vi "2898 Updated Secondary.vi"() -> (8 "Shooting Manual Override?":bool)   [LabVIEW 2011]
uses:
  Team Code/Robot Global Data.vi
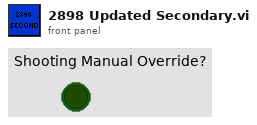
[diagram p1: front panel]
types:
  T1 = cluster{"Buttons":cluster{"A":bool, "B":bool, "X":bool, "Y":bool, "Left Bumper":bool, "Right Bumper":bool, "Back":bool, "Start":bool, "Left Thumbstick":bool, "Right Thumbstick":bool}, "Axes":cluster{"Left X ":dbl, "Left Y":dbl, "Triggers":dbl, "Right Stick X":dbl, "Right Stick Y":dbl, "D-Pad X":dbl}}
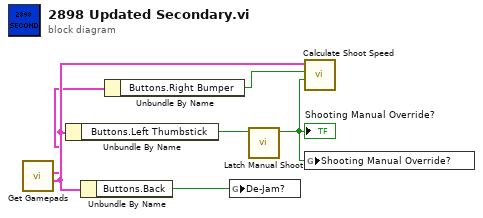
[diagram p0: block diagram]
diagram:
  n1 = call "Get Gamepads.vi"() -> ("Secondary"=w6:T1, "Driver"=w2:T1)  [unwired: 10 in]
  n2 = Unbundle By Name(w6) -> ("Buttons.Left Thumbstick"=w5:bool)
  n3 = Unbundle By Name(w6) -> ("Buttons.Back"=w3:bool)
  n4 = Unbundle By Name(w2) -> ("Buttons.Right Bumper"=w1:bool)
  n5 = global write "Robot Global Data.vi" "De-Jam?"(w3) -> ()
  n6 = call "Latch Manual Shoot.vi"("Input"=w5) -> ("Latched"=w4:bool)  [unwired: 10 in]
  "Shooting Manual Override?" <- w4
  n7 = call "Calculate Shoot Speed.vi"("Manual Override"=w4, "Driver Shoot"=w1, "Joystick"=w6) -> ()  [unwired: 9 in]
  n8 = global write "Robot Global Data.vi" "Shooting Manual Override?"(w4) -> ()
